vi "Calc Scale Factors_modded.vi"(2 "y axis attributes":T2 {"value 2" format="%.2f"; "value 1" format="%.2f"}, 3 "x axis attributes":T2 {"value 2" format="%.2f"; "value 1" format="%.2f"}) -> (0 "y scale factors":cluster{"a":dbl, "b":dbl, "log?":bool} {"b" format="%.2f"; "a" format="%.2f"}, 1 "x scale factors":cluster{"a":dbl, "b":dbl, "log?":bool} {"b" format="%.2f"; "a" format="%.2f"})   [LabVIEW 2018]
uses:
  fmt_prec_modded.ctl
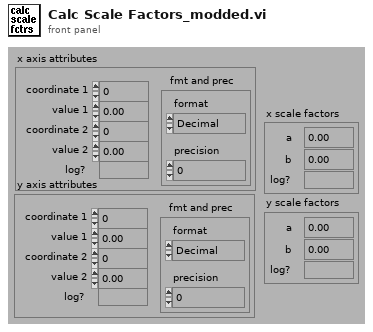
[diagram p1: front panel]
types:
  T1 = typedef "fmt_prec_modded.ctl" = cluster{"format":enum8{"Decimal", "Scientific", "Engineering", "Binary", "Octal", "Hex", "Timestamp"}, "precision":u8}
  T2 = cluster{"coordinate 1":i16, "value 1":dbl, "coordinate 2":i16, "value 2":dbl, "log?":bool, "fmt and prec":T1}
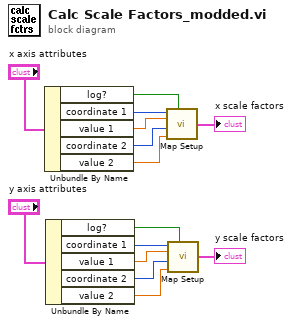
[diagram p0: block diagram]
diagram:
  n1 = Unbundle By Name("x axis attributes") -> ("log?"=w13:bool, "coordinate 1"=w10:i16, "value 1"=w9:dbl, "coordinate 2"=w12:i16, "value 2"=w11:dbl)
  n2 = Unbundle By Name("y axis attributes") -> ("log?"=w3:bool, "coordinate 1"=w6:i16, "value 1"=w7:dbl, "coordinate 2"=w4:i16, "value 2"=w5:dbl)
  n3 = call <vilib>:"Map Setup.vi"("coordinate 1"=w10, "value 1"=w9, "coordinate 2"=w12, "value 2"=w11, "log?(F)"=w13) -> ("scale factors"=→"x scale factors":cluster{"a":dbl, "b":dbl, "log?(F)":bool})
  n4 = call <vilib>:"Map Setup.vi"("coordinate 1"=w6, "value 1"=w7, "coordinate 2"=w4, "value 2"=w5, "log?(F)"=w3) -> ("scale factors"=→"y scale factors":cluster{"a":dbl, "b":dbl, "log?(F)":bool})
